vi "Read Calibrations+Settings from Dashboard.vi"   [LabVIEW 2014]
uses:
  <vilib>/Rock Robotics/Network Tables/SD Read Numeric Array.vi
  Global Variables/Calibrations.vi
  Global Variables/Settings.vi
types:
  T1 = cluster{"proportional gain (Kc)":dbl, "integral time (Ti, min)":dbl, "derivative time (Td, min)":dbl, "Maximum Value":dbl, "Minimum Value":dbl, "epsilon":dbl}
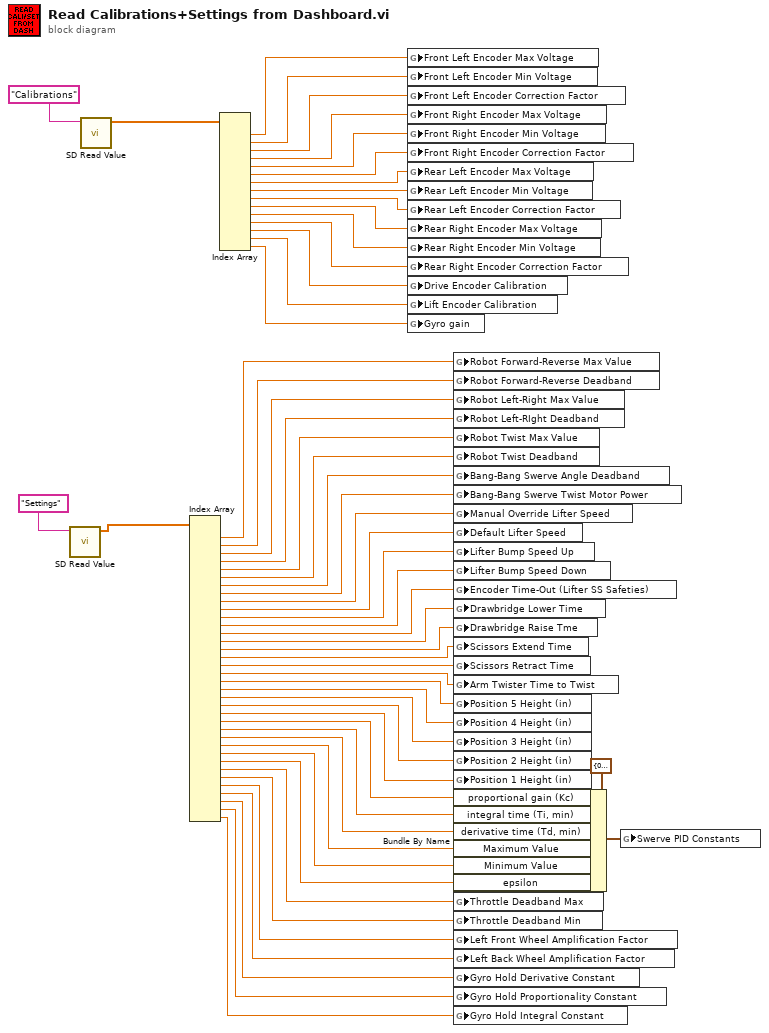
[diagram p0: block diagram]
diagram:
  n1 = call-poly <vilib>:"SD Read Value.vi"("Name"="Settings") -> ("Numeric Array"=w1:dbl[])  [unwired: 8 in, 2 out]
  n2 = call-poly <vilib>:"SD Read Value.vi"("Name"="Calibrations") -> ("Numeric Array"=w42:dbl[])  [unwired: 8 in, 2 out]
  n3 = Index Array(array=w1) -> (element #1=w11:dbl, element #2=w10:dbl, element #3=w37:dbl, element #4=w36:dbl, element #5=w35:dbl, element #6=w34:dbl, element #7=w33:dbl, element #8=w32:dbl, element #9=w31:dbl, element #10=w30:dbl, element #11=w29:dbl, element #12=w28:dbl, element #13=w27:dbl, element #14=w26:dbl, element #15=w25:dbl, element #16=w24:dbl, element #17=w23:dbl, element #18=w12:dbl, element #19=w22:dbl, element #20=w21:dbl, element #21=w20:dbl, element #22=w19:dbl, element #23=w18:dbl, element #24=w17:dbl, element #25=w9:dbl, element #26=w16:dbl, element #27=w15:dbl, element #28=w14:dbl, element #29=w13:dbl, element #30=w8:dbl, element #31=w7:dbl, element #32=w6:dbl, element #33=w5:dbl, element #34=w4:dbl, element #35=w3:dbl, element #36=w2:dbl)  [unwired: 36 in]
  n4 = Index Array(array=w42) -> (element #1=w57:dbl, element #2=w56:dbl, element #3=w55:dbl, element #4=w54:dbl, element #5=w53:dbl, element #6=w52:dbl, element #7=w51:dbl, element #8=w50:dbl, element #9=w49:dbl, element #10=w43:dbl, element #11=w48:dbl, element #12=w47:dbl, element #13=w45:dbl, element #14=w46:dbl, element #15=w44:dbl)  [unwired: 15 in]
  n5 = global write "Calibrations.vi" "Front Left Encoder Max Voltage"(w57) -> ()
  n6 = global write "Calibrations.vi" "Front Left Encoder Min Voltage"(w56) -> ()
  n7 = global write "Calibrations.vi" "Front Left Encoder Correction Factor"(w55) -> ()
  n8 = global write "Calibrations.vi" "Front Right Encoder Max Voltage"(w54) -> ()
  n9 = global write "Calibrations.vi" "Front Right Encoder Min Voltage"(w53) -> ()
  n10 = global write "Calibrations.vi" "Front Right Encoder Correction Factor"(w52) -> ()
  n11 = global write "Calibrations.vi" "Rear Left Encoder Max Voltage"(w51) -> ()
  n12 = global write "Calibrations.vi" "Rear Left Encoder Min Voltage"(w50) -> ()
  n13 = global write "Calibrations.vi" "Rear Left Encoder Correction Factor"(w49) -> ()
  n14 = global write "Calibrations.vi" "Rear Right Encoder Max Voltage"(w43) -> ()
  n15 = global write "Calibrations.vi" "Rear Right Encoder Min Voltage"(w48) -> ()
  n16 = global write "Calibrations.vi" "Rear Right Encoder Correction Factor"(w47) -> ()
  n17 = global write "Calibrations.vi" "Drive Encoder Calibration"(w45) -> ()
  n18 = global write "Calibrations.vi" "Lift Encoder Calibration"(w46) -> ()
  n19 = global write "Calibrations.vi" "Gyro gain"(w44) -> ()
  n20 = global write "Settings.vi" "Robot Forward-Reverse Max Value"(w11) -> ()
  n21 = global write "Settings.vi" "Robot Forward-Reverse Deadband"(w10) -> ()
  n22 = global write "Settings.vi" "Robot Left-Right Max Value"(w37) -> ()
  n23 = global write "Settings.vi" "Robot Left-RIght Deadband"(w36) -> ()
  n24 = global write "Settings.vi" "Robot Twist Max Value"(w35) -> ()
  n25 = global write "Settings.vi" "Robot Twist Deadband"(w34) -> ()
  n26 = global write "Settings.vi" "Bang-Bang Swerve Angle Deadband"(w33) -> ()
  n27 = global write "Settings.vi" "Bang-Bang Swerve Twist Motor Power"(w32) -> ()
  n28 = global write "Settings.vi" "Manual Override Lifter Speed"(w31) -> ()
  n29 = global write "Settings.vi" "Default Lifter Speed"(w30) -> ()
  n30 = global write "Settings.vi" "Lifter Bump Speed Up"(w29) -> ()
  n31 = global write "Settings.vi" "Lifter Bump Speed Down"(w28) -> ()
  n32 = global write "Settings.vi" "Encoder Time-Out (Lifter SS Safeties)"(w27) -> ()
  n33 = global write "Settings.vi" "Drawbridge Lower Time"(w26) -> ()
  n34 = global write "Settings.vi" "Drawbridge Raise Tme"(w25) -> ()
  n35 = global write "Settings.vi" "Scissors Extend Time"(w24) -> ()
  n36 = global write "Settings.vi" "Scissors Retract Time"(w23) -> ()
  n37 = global write "Settings.vi" "Arm Twister Time to Twist"(w12) -> ()
  n38 = global write "Settings.vi" "Position 5 Height (in)"(w22) -> ()
  n39 = global write "Settings.vi" "Position 4 Height (in)"(w21) -> ()
  n40 = global write "Settings.vi" "Position 3 Height (in)"(w20) -> ()
  n41 = global write "Settings.vi" "Position 2 Height (in)"(w19) -> ()
  n42 = global write "Settings.vi" "Position 1 Height (in)"(w18) -> ()
  n43 = Bundle By Name(cluster=T1 {"proportional gain (Kc)"=0.025, "integral time (Ti, min)"=0.0, "derivative time (Td, min)"=0.0005, "Maximum Value"=0.0005, "Minimum Value"=0.0005, "epsilon"=0.0005} ("Swerve PID Constants"), "proportional gain (Kc)"=w17, "integral time (Ti, min)"=w9, "derivative time (Td, min)"=w16, "Maximum Value"=w15, "Minimum Value"=w14, "epsilon"=w13) -> (w39:T1)
  n44 = global write "Settings.vi" "Throttle Deadband Max"(w8) -> ()
  n45 = global write "Settings.vi" "Throttle Deadband Min"(w7) -> ()
  n46 = global write "Settings.vi" "Left Front Wheel Amplification Factor"(w6) -> ()
  n47 = global write "Settings.vi" "Left Back Wheel Amplification Factor"(w5) -> ()
  n48 = global write "Settings.vi" "Gyro Hold Derivative Constant"(w4) -> ()
  n49 = global write "Settings.vi" "Gyro Hold Proportionality Constant"(w3) -> ()
  n50 = global write "Settings.vi" "Gyro Hold Integral Constant"(w2) -> ()
  n51 = global write "Settings.vi" "Swerve PID Constants"(w39) -> ()
